vi "CorrectionParameters.vi"(0 "Aberration Correction On":bool, 1 "Aberration Correction":sgl[](array[numeric])=array[262144 elements], 3 "Polynomial Order":i32=3 min=3 max=7 step=1, 5 "SaveAmplitudes":bool, 6 "Polynomial Coefficients":sgl[](array[numeric])=[1.0, 0.0, 0.0, 0.0, 0.0, 0.0, 0.0, 0.0, 0.0, 0.0, 0.0, 0.0, 0.0, 0.0, 0.0, 0.0, 0.0, 0.0, 0.0, 0.0, 0.0, 0.0, 0.0, 0.0, 0.0, 0.0, 0.0, 0.0, 0.0, 0.0, 0.0, 0.0, 0.0, 0.0, 0.0, 0.0, 0.0, 0.0, 0.0, 0.0, 0.0, 0.0, 0.0, 0.0, 0.0, 0.0, 0.0, 0.0, 0.0, 0.0, 0.0, 0.0, 0.0, 0.0, 0.0, 0.0, 0.0, 0.0, 0.0, 0.0, 0.0, 0.0, 0.0, 0.0, 0.0, 0.0, 0.0, 0.0, 0.0, 0.0, 0.0, 0.0, 0.0, 0.0, 0.0, 0.0, 0.0, 0.0, 0.0, 0.0, 0.0, 0.0, 0.0, 0.0, 0.0, 0.0, 0.0, 0.0, 0.0, 0.0, 0.0, 0.0, 0.0, 0.0, 0.0, 0.0, 0.0, 0.0, 0.0, 0.0, 0.0, 0.0, 0.0, 0.0, 0.0, 0.0, 0.0, 0.0, 0.0, 0.0, 0.0, 0.0, 0.0, 0.0, 0.0, 0.0, 0.0, 0.0, 0.0, 0.0], 7 "useLUT":bool, 9 "DCborderWidth":i32, 10 "Use polynomial LUT":bool, 11 "error in":errorcluster, 12 "LUT":i8[](array[numeric]), 14 "AlphaRPC":sgl) -> (4 "CUDA Return":i32, 15 "error out":errorcluster)   [LabVIEW 2011]
uses:
  GenerateHologramCUDA.dll
panel:
  out "LUTPolCoeff":sgl[](array[numeric])
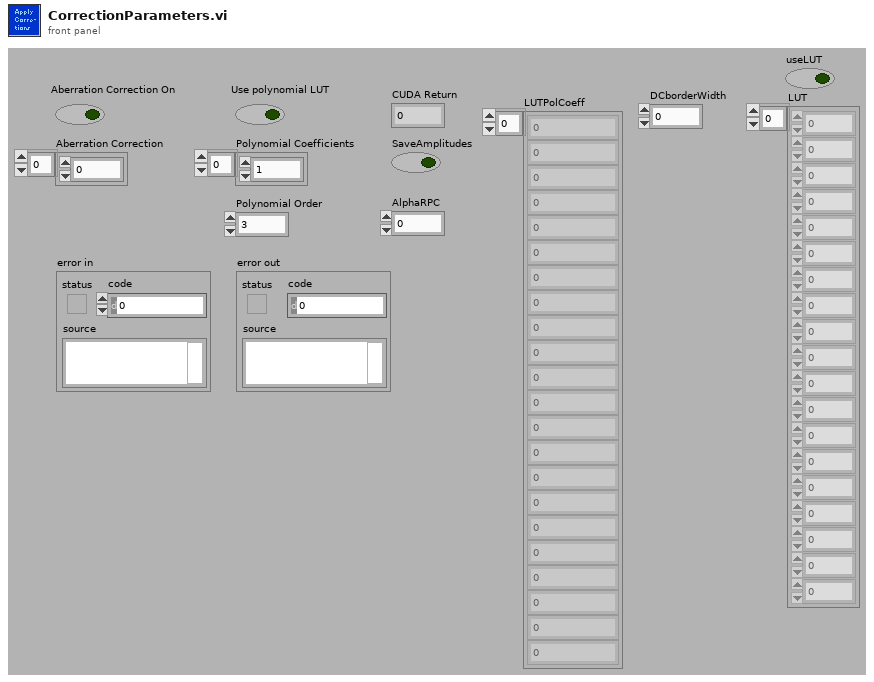
[diagram p1: front panel]
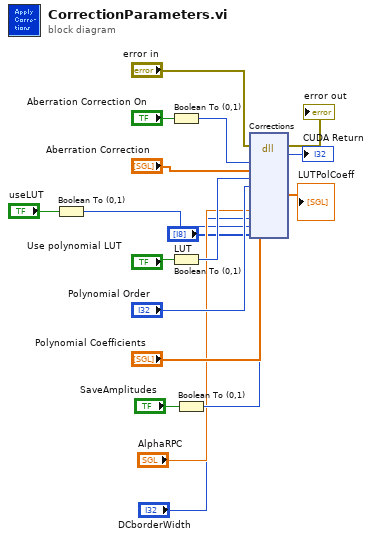
[diagram p0: block diagram]
diagram:
  n1 = Boolean To (0,1)(Boolean="useLUT") -> (0, 1=w2:i16)
  n2 = Boolean To (0,1)(Boolean="Aberration Correction On") -> (0, 1=w9:i16)
  n3 = Boolean To (0,1)(Boolean="Use polynomial LUT") -> (0, 1=w14:i16)
  n4 = Boolean To (0,1)(Boolean="SaveAmplitudes") -> (0, 1=w6:i16)
  n5 = dll-call lib="C:/Users/Martin/Dropbox/GU/CUDA/GenerateHologramCUDA/LabVIEW/GenerateHologramCUDA.dll" fn="Corrections"(error in="error in", "useAberrationCorrection"=w9, "AberrationCorrection"="Aberration Correction", "useLUTPol"=w14, "PolOrder"="Polynomial Order", "LUTPolCoeff"="Polynomial Coefficients", "SaveAmplitudes"=w6, "AlphaRPC"="AlphaRPC", "DCborderWidth"="DCborderWidth", "useLUT"=w2, "LUT"="LUT") -> (error out=→"error out":errorcluster, "return type"=→"CUDA Return":i32, "LUTPolCoeff"=→"LUTPolCoeff":sgl[])  [unwired: 11 in, 1 out]
